vi "Calculate Accuracy.vi"(8 "Error In":errorcluster, 9 "CAL_DUT_CONT":i32[](array[numeric]), 10 "CAL_DUT_ERR":i32[](array[numeric])) -> (0 "Error Out":errorcluster, 1 "Revolution Index":i32[](array[numeric]), 2 "Accuracy [Degree]":dbl[](array[numeric]), 3 "Accuracy [Bit]":dbl[](array[numeric]))   [LabVIEW 2019]
doc: "Berechnung der Kalibriergenauigkeit pro Umdrehung. Gibt zusätzlich die Indexpunkte für die Umdrehungen im Array an\n\nParameters:\n- CAL_DUT_ERR (Numeric Array)\n- CAL_DUT_CONT (Numeric Array)\n- Accuracy [Bit] (Numeric)\n- Accuracy [Degree] (Numeric)\n- Revolution Index (i32 Array)\n- Error In/ Error Out"
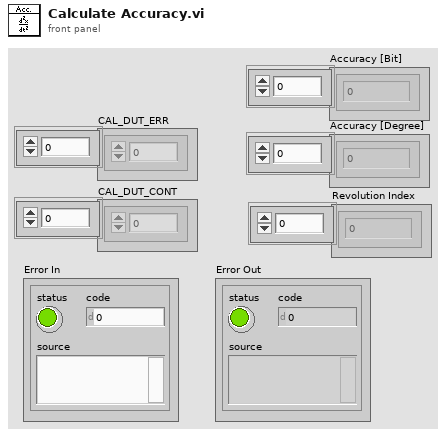
[diagram p1: front panel]
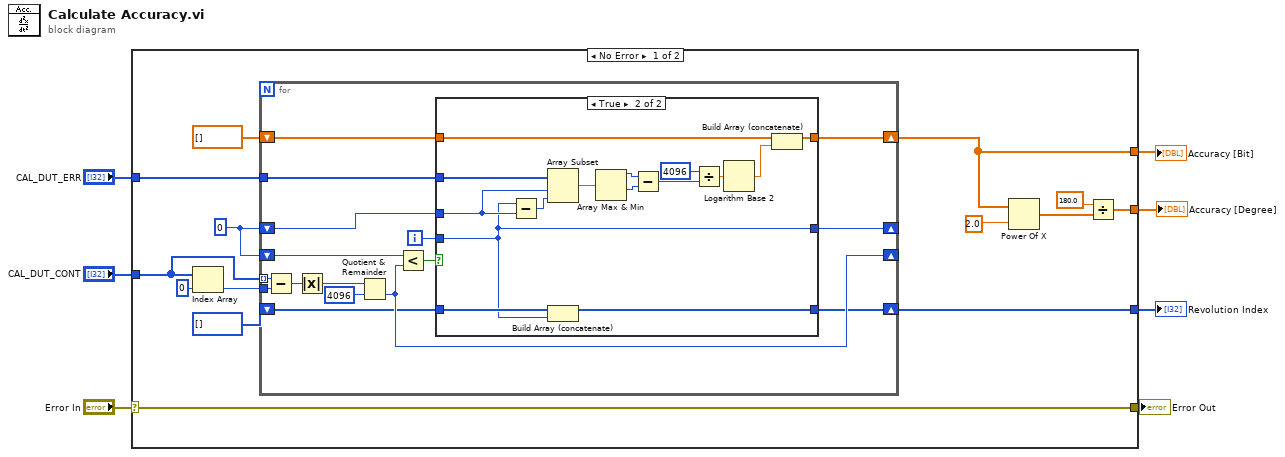
[diagram p0: block diagram]
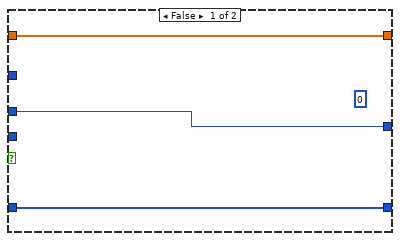
[diagram p2: hidden frame]
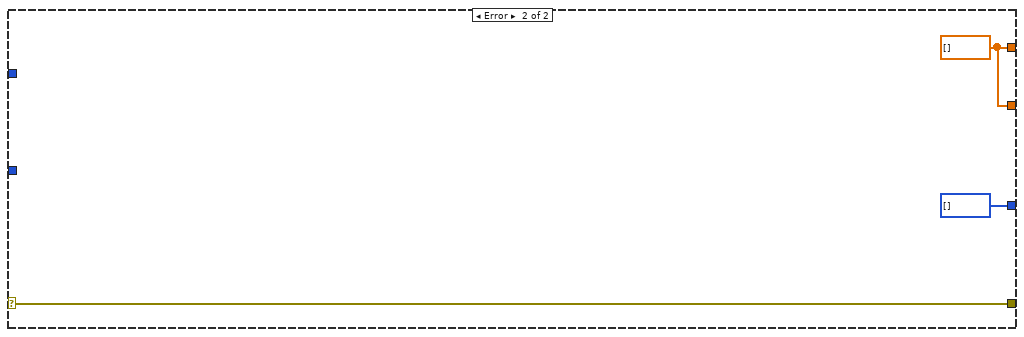
[diagram p3: hidden frame]
diagram:
  n1 = case shown="No Error" "Error In" {
    selector: "Error In" -> [w16 w58]
    tunnel: "CAL_DUT_CONT" -> [w13 _]
    tunnel: "CAL_DUT_ERR" -> [w17 _]
    tunnel: [w16 w58] -> w4
    tunnel: [w8 w56] -> w3
    tunnel: [w14 w56] -> w1
    tunnel: [w11 i32[] []] -> w2
    frame No Error {
      w20 = 0
      n2 = Index Array(array=w13, index=0) -> (element=w21:i32)
      n3 = for {
        shift-right: [w29] -> _
        shift-left: w20 -> [w30]
        shift-right: [w35] -> _
        shift-left: w20 -> [w34]
        shift-right: [w31] -> w8
        shift-left: dbl[] [] -> [w32]
        tunnel: w17 -> [w26]
        tunnel: w21 -> [w25]
        tunnel: w13 -> [w24] mode=indexing
        shift-right: [w23] -> w11
        shift-left: i32[] [] -> [w22]
        i -> [w36]
        n4 = Subtract(x=w24, y=w25) -> (x-y=w28:i32)
        n5 = Absolute Value(x=w28) -> (abs(x)=w27:i32)
        n6 = Quotient & Remainder(x=w27, y=4096) -> (floor(x/y)=w29:i32)  [unwired: 1 out]
        n7 = Less?(x=w30, y=w29) -> (x < y?=w33:bool)
        n8 = case shown="True" w33 {
          tunnel: w36 -> [_ w42]
          tunnel: [w40 w42] -> w35
          tunnel: w34 -> [w40 w55]
          tunnel: w32 -> [w39 w49]
          tunnel: [w39 w50] -> w31
          tunnel: w26 -> [_ w45]
          tunnel: [w38 w41] -> w23
          tunnel: w22 -> [w38 w43]
          frame False {
            (unwired) 0
          }
          frame True {
            n9 = Subtract(x=w42, y=w55) -> (x-y=w54:i32)
            n10 = Array Subset(array=w45, index=w55, length=w54) -> (w48:i32[])
            n11 = Build Array (concatenate)(w43, w42) -> (w41:i32[])
            n12 = Array Max & Min(array=w48) -> (max value=w46:i32, min value=w47:i32)  [unwired: 2 out]
            n13 = Subtract(x=w46, y=w47) -> (x-y=w44:i32)
            n14 = Divide(x=4096, y=w44) -> (x/y=w52:dbl)
            n15 = Logarithm Base 2(1:w52) -> (0:w51:dbl)
            n16 = Build Array (concatenate)(w49, w51) -> (w50:dbl[])
          }
        }
      }
      n17 = Power Of X(1:2.0 ("x"), 2:w8) -> (0:w10:dbl[])
      n18 = Divide(x=180.0, y=w10) -> (x/y=w14:dbl[])
    }
    frame Error {
      w56 = dbl[] []
    }
  }
  "Error Out" <- w4
  "Revolution Index" <- w2
  "Accuracy [Bit]" <- w3
  "Accuracy [Degree]" <- w1
